vi "Reset_Instr.vi"(8 "error in (no error)":errorcluster caption="entrée d'erreur (pas d'erreur)", 11 "Class Instrument Multimeter en entrée":refnum<class "Class Instrument Schielding_Box.lvclass">) -> (0 "error out":errorcluster caption="sortie d'erreur", 3 "Class Instrument Multimeter en sortie":refnum<class "Class Instrument Schielding_Box.lvclass">)   [LabVIEW 2020, in "Library Instrument & Equipement.lvlib" / "Library Instruments.lvlib" / "Class Instrument Schielding_Box.lvclass"]
uses:
  Class Instrument Schielding_Box.lvclass
  Class Instrument Schielding_Box.lvclass/Class Instrument Schielding_Box.ctl
  Instrument (Default)/Class Instrument (Default).lvclass
  Shielding box/Class Shielding box (Default)/Class Shielding_ Box (Default).lvclass
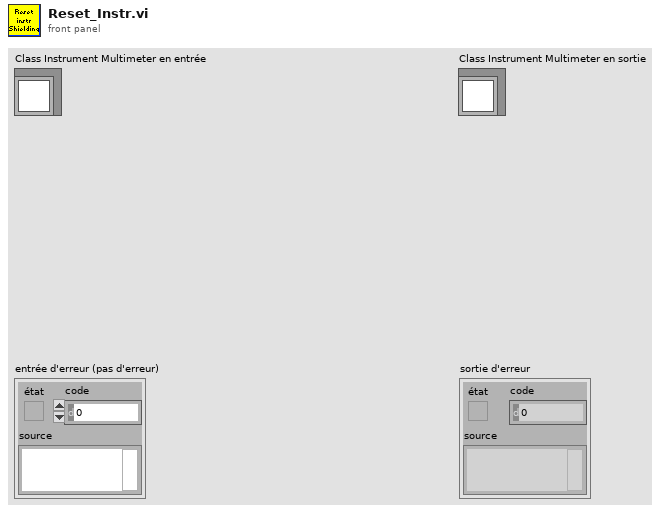
[diagram p1: front panel]
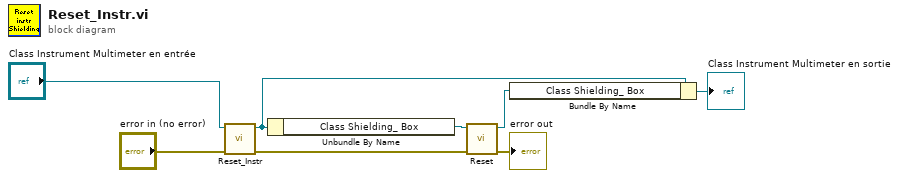
[diagram p0: block diagram]
diagram:
  n1 = call-parent "Reset_Instr.vi"("error in (no error)"="error in (no error)", "Class Instrument (Default) en entrée"="Class Instrument Multimeter en entrée") -> ("error out"=w3:errorcluster, "Class Instrument (Default) en sortie"=w6:refnum<class "Class Instrument Schielding_Box.lvclass">)  [unwired: 8 in]
  n2 = Unbundle By Name(w6) -> ("Class Shielding_ Box"=w4:refnum<class "Class Shielding_ Box (Default).lvclass">)
  n3 = call-dynamic "Reset.vi"("error in (no error)"=w3, "Class Shielding_ Box (Default) en entrée"=w4) -> ("error out"=→"error out":errorcluster, "Class Shielding_ Box (Default) en sortie"=w1:refnum<class "Class Shielding_ Box (Default).lvclass">)  [unwired: 8 in]
  n4 = Bundle By Name(cluster=w6, "Class Shielding_ Box"=w1) -> (→"Class Instrument Multimeter en sortie":refnum<class "Class Instrument Schielding_Box.lvclass">)
